vi "Periodic Tasks.vi"() -> ()   [LabVIEW 2019]
doc: "This VI runs in parallel to other tasks. It can contain as many user-defined periodic loops as you need. These can carry out PID or other sorts of timed response."
uses:
  <vilib>/Rock Robotics/Network Tables/NT Read Number.vi
  Global Data.vi
  Refnums.vi
  <vilib>/Rock Robotics/Network Tables/NT Write String.vi
  <vilib>/Rock Robotics/Network Tables/NT Read String.vi
  <vilib>/Rock Robotics/WPI/ThirdParty/Phoenix-LabVIEW/Motor Controller/Controls/CTRE_Phoenix_MotorControl_ControlMode.ctl
  <vilib>/Rock Robotics/WPI/ThirdParty/Phoenix-LabVIEW/Motor Controller/Get/CTRE_Phoenix_MotorController_GetQuadratureData.vi
panel:
  in  "Numeric":dbl
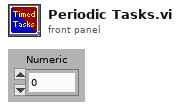
[diagram p1: front panel]
types:
  T1 = typedef "WPI_DriverStationRobotMode2.ctl" = enum16{"Autonomous Disabled", "Autonomous Enabled", "Teleop Disabled", "Teleop Enabled", "Disconnected", "Finish", "Test Disabled", "Test Enabled", "Emergency Stopped"}
  T2 = typedef "CTRE_Phoenix_MotorControl_ControlMode.ctl" = u16
  T3 = typedef "WPI_RobotDriveDevRef.ctl" = cluster{"DevStatus":errorcluster, "Motors[]":T4[], "Square Inputs":bool, "Max Output":dbl}
  T4 = typedef "WPI_MotorControlDeviceRef.ctl" = cluster{"DeviceStatus":errorcluster, "Type":T5, "PWM":cluster{"PWM Channel":T6, "DeadBand":T7}, "CAN":cluster{"Device Number":u8, "SetOutput VI Ref":variant, "GetOutput VI Ref":variant, "Enable VI Ref":variant, "Disable VI Ref":variant, "Data":variant}, "Invert":bool, "DIO PWM":cluster{"PWM \"Enable\" Channel":T6, "DIOChannel":T8, "PWM Rate":dbl}}
  T5 = typedef "WPI_MotorControlType.ctl" = enum16{"PWM", "CAN", "DIO PWM"}
  T6 = typedef "FPGA_DIOPWMChannel.ctl" = enum8{"PWM 0", "PWM 1", "PWM 2", "PWM 3", "PWM 4", "PWM 5", "PWM 6", "PWM 7", "PWM 8", "PWM 9", "PWM MXP 0", "PWM MXP 1", "PWM MXP 2", "PWM MXP 3", "PWM MXP 4", "PWM MXP 5", "PWM MXP 6", "PWM MXP 7", "PWM MXP 8", "PWM MXP 9", "Invalid"}
  T7 = typedef "WPI_PWMDeadband.ctl" = cluster{"Name":string, "maxPositivePwm":i32, "minPositivePwm":i32, "centerPwm":i32, "maxNegativePwm":i32, "minNegativePwm":i32, "angularRange":u16}
  T8 = typedef "FPGA_DIOChannel.ctl" = enum8{"DIO 0", "DIO 1", "DIO 2", "DIO 3", "DIO 4", "DIO 5", "DIO 6", "DIO 7", "DIO 8", "DIO 9", "DIO MXP 0", "DIO MXP 1", "DIO MXP 2", "DIO MXP 3", "DIO MXP 4", "DIO MXP 5", "DIO MXP 6", "DIO MXP 7", "DIO MXP 8", "DIO MXP 9", "DIO MXP 10", "DIO MXP 11", "DIO MXP 12", "DIO MXP 13", "DIO MXP 14", "DIO MXP 15", "SPI Port CS1", "SPI Port CS2", "SPI Port CS3", "SPI Port MISO", "SPI Port MOSI", "Invalid"}
  T9 = cluster{"ROBOT_DRIVE":T3, "TURRET":T4, "SHOOTER_MASTER":T4, "HOPPER":T4, "INDEXER":T4, "INTAKE":T4, "CLIMBER_WINCH":T4, "CLIMBER_ARM":T4, "SHOOTER_ANGLE":T4, "SHOOTER_SLAVE":T4, "AGITATOR":T4, "AGITATOR OLD":T4, "LEFT_MASTER":T4, "RIGHT_MASTER":T4}
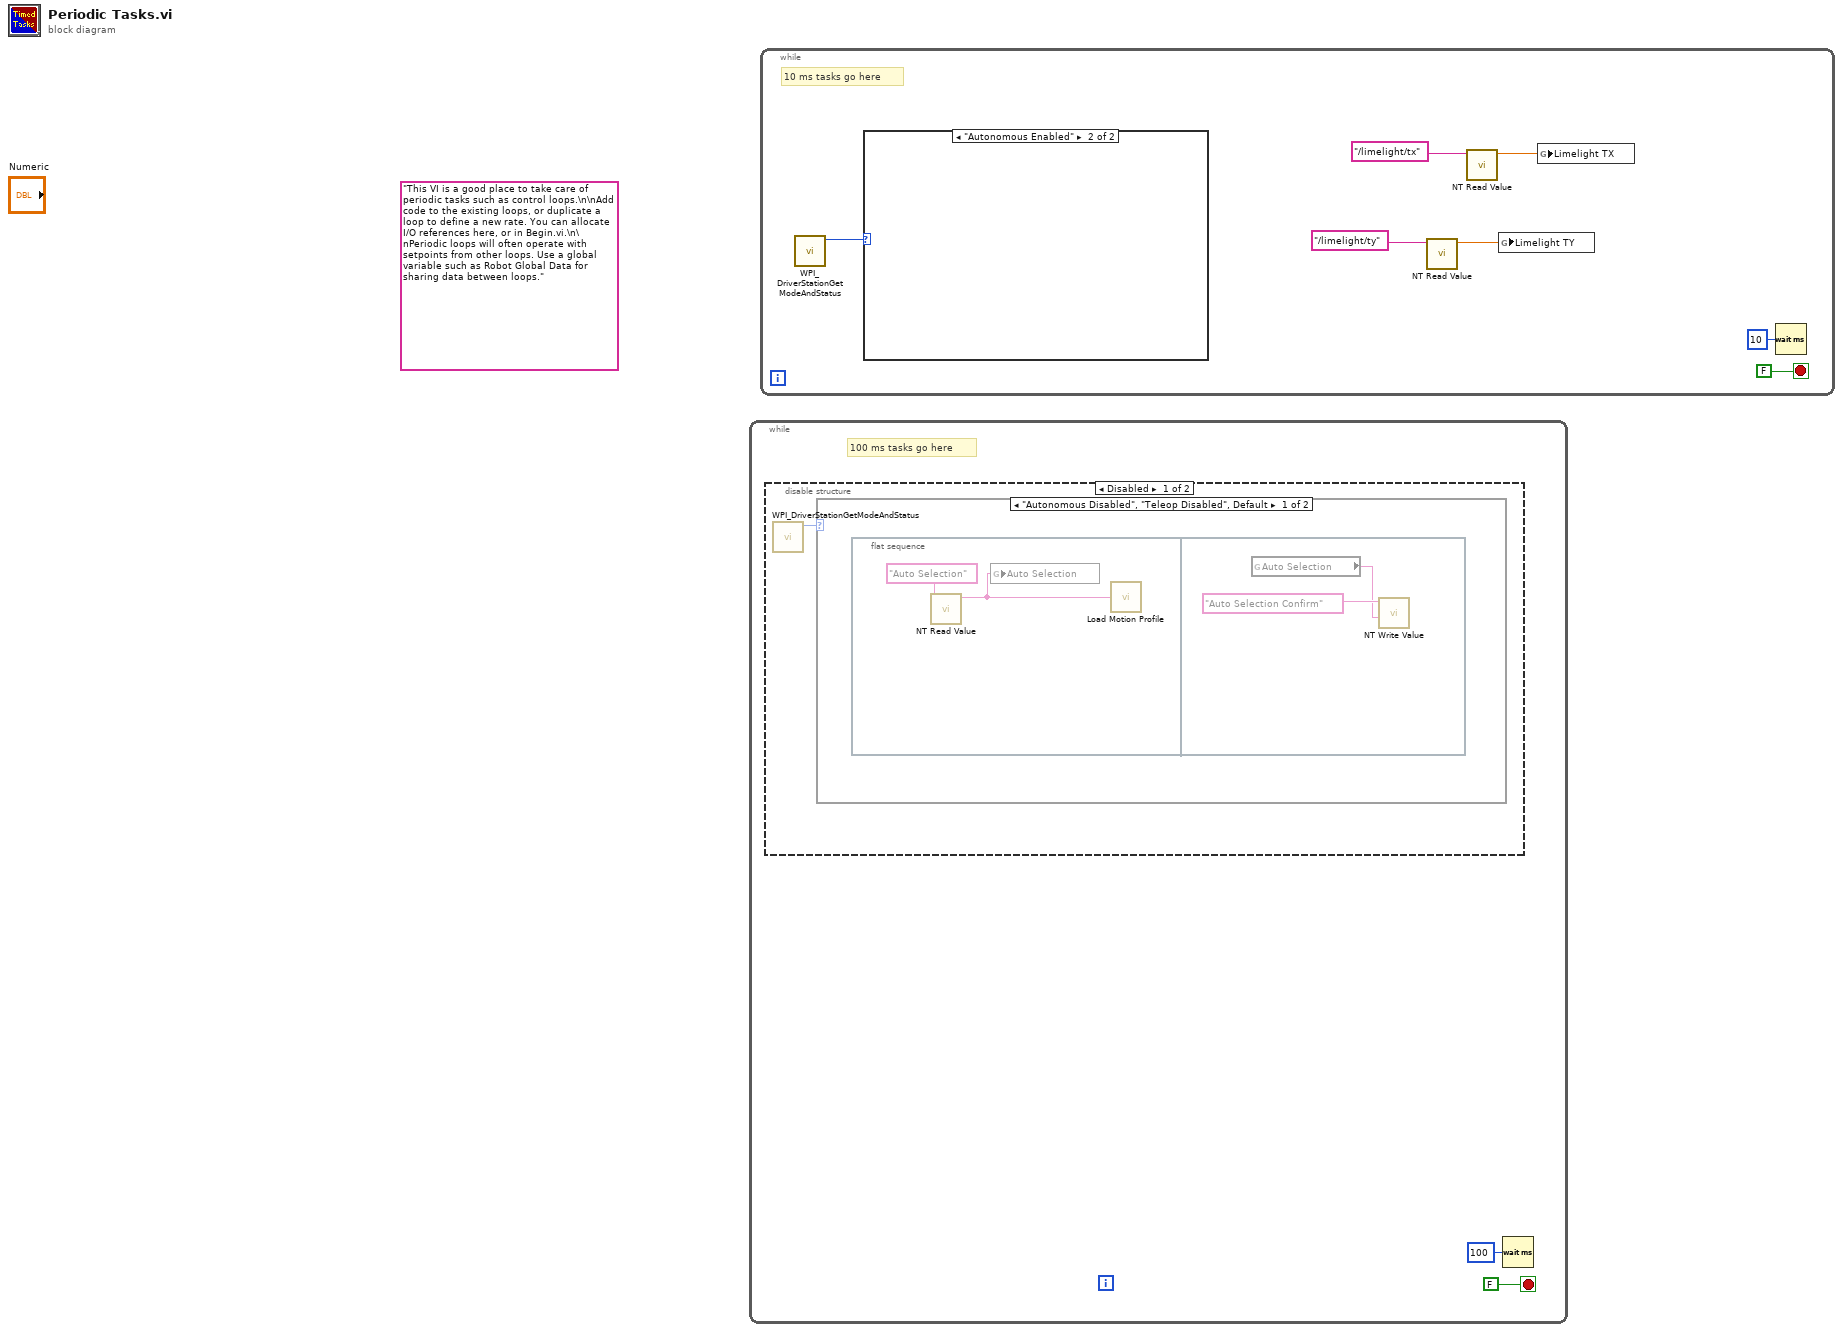
[diagram p0: block diagram]
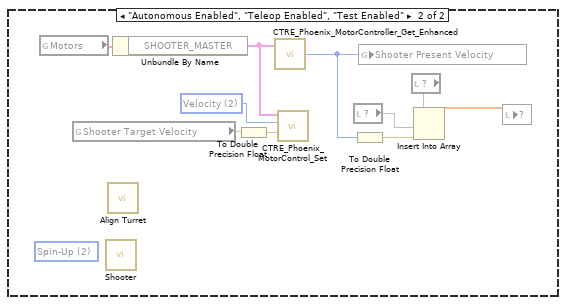
[diagram p2: hidden frame]
diagram:
  (unwired) "This VI is a good place to take care of periodic tasks such as control loops.\n\nAdd code to the existing loops, or duplicate a loop to define a new rate. You can allocate I/O references here, or in Begin.vi.\n\nPeriodic loops will often operate with setpoints from other loops. Use a global variable such as Robot Global Data for sharing data between loops."
  n1 = while {
    stop <- FALSE stop-if-true
    # "100 ms tasks go here"
    n2 = disable-structure shown="Disabled" {
      frame Disabled {
        n3 = call <vilib>:"WPI_DriverStationGetModeAndStatus.vi"() -> ("Robot Mode"=w3:T1)  [unwired: 10 in, 1 out]
        n4 = case shown="\"Autonomous Disabled\", \"Teleop Disabled\", Default" w3 {
          frame "Autonomous Disabled", "Teleop Disabled", Default {
            n5 = flat-sequence {
              frame #0 {
                n6 = call-poly <vilib>:"NT Read Value.vi"("Name"="Auto Selection") -> ("String"=w4:string)  [unwired: 9 in, 1 out]
                n7 = global write "Global Data.vi" "Auto Selection"(w4) -> ()
                n8 = call "Load Motion Profile.vi"("Left File Path"=w4) -> ()  [unwired: 4 in]
              }
              frame #1 {
                n9 = global read "Global Data.vi" "Auto Selection"() -> (w6:string)
                n10 = call-poly <vilib>:"NT Write Value.vi"("String"=w6, "Name"="Auto Selection Confirm") -> ()  [unwired: 9 in, 1 out]
              }
            }
          }
          frame "Autonomous Enabled", "Teleop Enabled", "Test Enabled" {
            (unwired) u16 2 items=["Stop", "Shoot", "Spin-Up"] ("Shoot or Spin")
            w15 = T2 2 items=["PercentOutput"=0, "Position"=1, "Velocity"=2, "Current"=3, "Follower"=5, "MotionProfile"=6, "MotionMagic"=7, "MotionProfileArc"=10, "Disabled"=15] ("Control Mode")
            n11 = global read "Refnums.vi" "Motors"() -> (w17:T9)
            n12 = global read "Global Data.vi" "Shooter Target Velocity"() -> (w14:dbl)
            n13 = call "Shooter.vi"() -> ()  [unwired: 12 in]
            n14 = call "Align Turret.vi"() -> ()  [unwired: 12 in]
            n15 = Unbundle By Name(w17) -> ("SHOOTER_MASTER"=w16:T4)
            n16 = To Double Precision Float(number=w14) -> (double precision float=w13:dbl)
            n17 = call-poly <vilib>:"CTRE_Phoenix_MotorController_Get_Enhanced.vi"("PhoenixMotorControlDevRef"=w16) -> ("Quadrature Velocity"=w10:i32)  [unwired: 11 in, 3 out]
            n18 = call <vilib>:"CTRE_Phoenix_MotorControl_Set.vi"("Output"=w13, "Control Mode"=w15, "PhoenixMotorControlDevRef"=w16) -> ()  [unwired: 7 in, 2 out]
            n19 = local read item#-1() -> (w8)
            n20 = To Double Precision Float(number=w10) -> (double precision float=w9:dbl)
            n21 = global write "Global Data.vi" "Shooter Present Velocity"(w10) -> ()
            n22 = local read item#-1() -> (w12)
            n23 = Insert Into Array(array=w12, index=w8, new element=w9) -> (w11:dbl[])
            n24 = local write item#-1(w11) -> ()
          }
        }
      }
      frame Enabled {
      }
    }
    n25 = Wait (ms)(milliseconds to wait=u32 100) -> ()  [unwired: 1 out]
  }
  n26 = while {
    stop <- FALSE stop-if-true
    # "10 ms tasks go here"
    n27 = call <vilib>:"WPI_DriverStationGetModeAndStatus.vi"() -> ("Robot Mode"=w22:T1)  [unwired: 10 in, 1 out]
    n28 = case shown="\"Autonomous Enabled\"" w22 {
      frame "Autonomous Disabled", Default {
      }
      frame "Autonomous Enabled" {
      }
    }
    n29 = call-poly <vilib>:"NT Read Value.vi"("Name"="/limelight/ty") -> ("Numeric"=w18:dbl)  [unwired: 9 in, 1 out]
    n30 = call-poly <vilib>:"NT Read Value.vi"("Name"="/limelight/tx") -> ("Numeric"=w20:dbl)  [unwired: 9 in, 1 out]
    n31 = global write "Global Data.vi" "Limelight TY"(w18) -> ()
    n32 = global write "Global Data.vi" "Limelight TX"(w20) -> ()
    n33 = Wait (ms)(milliseconds to wait=u32 10) -> ()  [unwired: 1 out]
  }
